vi "svc_Split Waveform (Index).vi"(8 "error in (no error)":errorcluster, 10 "index":i32, 11 "waveform in":waveform(dbl)) -> (0 "error out":errorcluster, 2 "second waveform out":waveform(dbl), 3 "first waveform out":waveform(dbl))   [LabVIEW 2017]
doc: "Divides the <B>waveform in</B> at <B>start index</B> and returns the two waveforms."
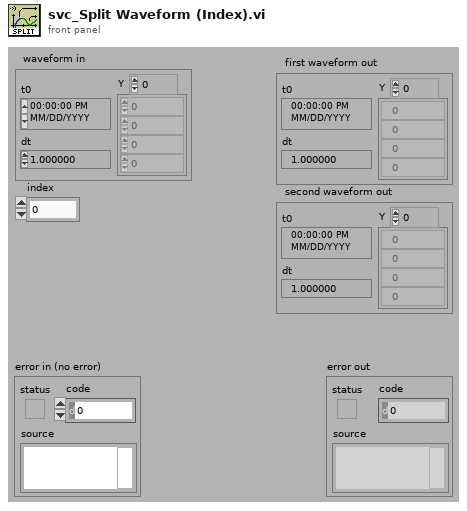
[diagram p1: front panel]
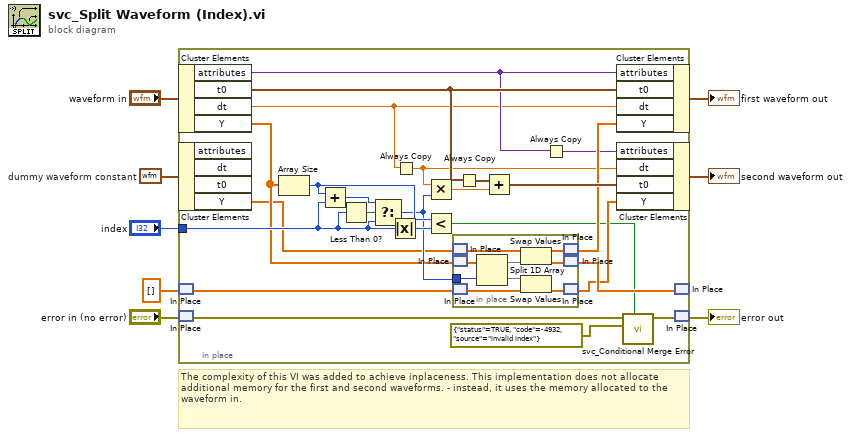
[diagram p0: block diagram]
diagram:
  w5 = waveform(dbl) {"t0"=timestamp(0 s since 1904-01-01), "dt"=1.0, "Y"=[]}  # dummy waveform constant
  # "The complexity of this VI was added to achieve inplaceness. This implementation does not allocate additional memory for the first and second waveforms. - instead, it uses the memory allocated to the waveform in."
  n1 = in-place {
    in-place-border: "index" -> [w26]
    n2 = in-place-cluster #1("waveform in") -> ("attributes"=w24:variant, "t0"=w31:timestamp, "dt"=w19:dbl, "Y"=w22:dbl[])
    n3 = in-place-cluster #2(w5) -> ("Y"=w16:dbl[])  [unwired: 3 out]
    n4 = in-place-match #3(dbl[] [] ("Y")) -> (w18:dbl[])
    n5 = in-place-match #4("error in (no error)") -> (w14:errorcluster)
    n6 = Array Size(array=w22) -> (size(s)=w27:i32)
    n7 = Add(x=w27, y=w26) -> (x+y=w29:i32)
    n8 = Less Than 0?(x=w26) -> (x < 0?=w30:bool)
    n9 = Select(t=w29, s=w30, f=w26) -> (s? t:f=w25:i32)
    n10 = Absolute Value(x=w26) -> (abs(x)=w28:i32)
    n11 = Always Copy(1:w19) -> (0:w10:dbl)
    n12 = Multiply(x=w10, y=w25) -> (x*y=w32:dbl)
    n13 = Less?(x=w27, y=w28) -> (x < y?=w12:bool)
    n14 = in-place {
      in-place-border: w25 -> [w41]
      n15 = in-place-match #5(w16) -> (w35:dbl[])
      n16 = in-place-match #6(w22) -> (w40:dbl[])
      n17 = in-place-match #7(w18) -> (w39:dbl[])
      n18 = Split 1D Array(array=w40, index=w41) -> (first subarray=w36:dbl[], second subarray=w38:dbl[])
      n19 = Swap Values(12:w35, 14:w36) -> (1:w34:dbl[], 3:w33:dbl[])  [unwired: 1 in]
      n20 = Swap Values(12:w38, 14:w39) -> (3:w37:dbl[])  [unwired: 1 in, 1 out]
      n21 = in-place-match #5(w34) -> (w21:dbl[])
      n22 = in-place-match #6(w33) -> (w20:dbl[])
      n23 = in-place-match #7(w37) -> (w17:dbl[])
    }
    n24 = Always Copy(1:w31) -> (0:w9:timestamp)
    n25 = Add(x=w9, y=w32) -> (x+y=w23:timestamp)
    n26 = Always Copy(1:w24) -> (0:w11:variant)
    n27 = in-place-cluster #1("attributes"=w24, "t0"=w31, "dt"=w19, "Y"=w21) -> (→"first waveform out":waveform(dbl))
    n28 = in-place-cluster #2("attributes"=w11, "dt"=w10, "t0"=w23, "Y"=w17) -> (→"second waveform out":waveform(dbl))
    n29 = call <vilib>:"svc_Conditional Merge Error.vi"("merge"=w12, "new error"=errorcluster {"status"=TRUE, "code"=-4932, "source"="invalid index"} ("error out"), "error in (no error)"=w14) -> ("error out"=w13:errorcluster)  [unwired: 8 in]
    n30 = in-place-match #3(w20) -> ()  [unwired: 1 out]
    n31 = in-place-match #4(w13) -> (→"error out":errorcluster)
  }
